vi "Update_Results_file_copies.vi"(2 "Raw data option":enum16{"Save raw data", "Raw data not saved"}(ring), 4 "Raw data file":path, 5 "Results file":path) -> ()   [LabVIEW 2022 SP3]
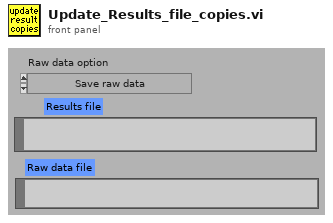
[diagram p1: front panel]
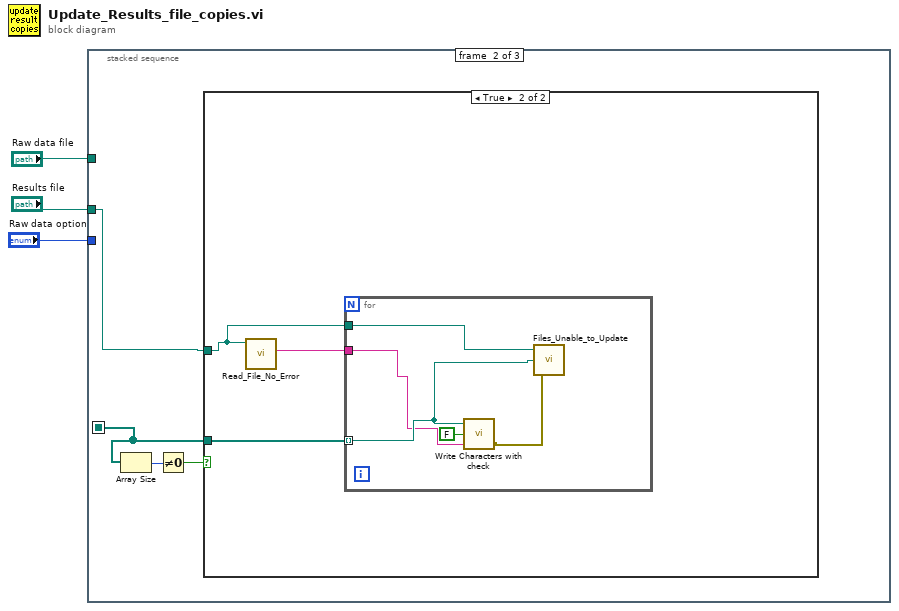
[diagram p0: block diagram]
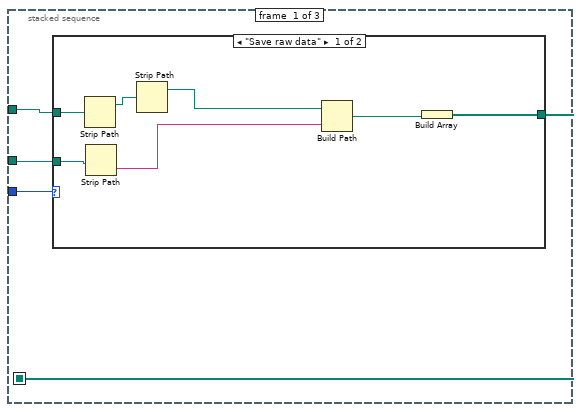
[diagram p2: hidden frame]
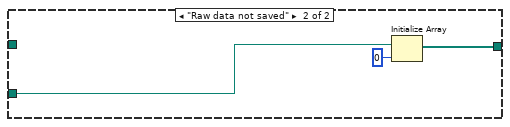
[diagram p3: hidden frame]
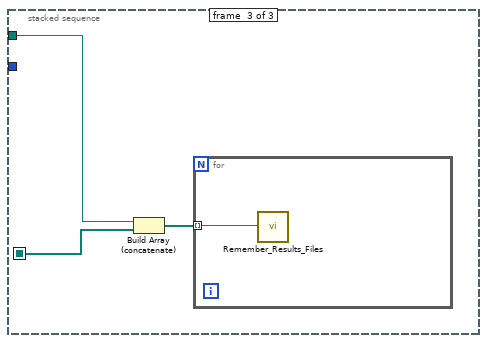
[diagram p5: hidden frame]
diagram:
  n1 = stacked-sequence {
    seq-local: [w4 _ _] -> [_ w18 w30]
    tunnel: "Results file" -> [w7 w19 w31]
    tunnel: "Raw data file" -> [w6 _ _]
    tunnel: "Raw data option" -> [w5 _ _]
    frame #0 {
      n2 = case shown="\"Save raw data\"" w5 {
        tunnel: w6 -> [w12 _]
        tunnel: w7 -> [w13 w15]
        tunnel: [w14 w16] -> w4
        frame "Save raw data" {
          n3 = Strip Path(path=w12) -> (stripped path=w9:path)  [unwired: 1 out]
          n4 = Strip Path(path=w13) -> (name=w11:string)  [unwired: 1 out]
          n5 = Strip Path(path=w9) -> (stripped path=w8:path)  [unwired: 1 out]
          n6 = Build Path(base path=w8, name or relative path=w11) -> (appended path=w10:path)
          n7 = Build Array(w10) -> (w14:path[])
        }
        frame "Raw data not saved" {
          n8 = Initialize Array(w15, 0 ("Dimension Size")) -> (w16:path[])
        }
      }
    }
    frame #1 {
      n9 = Array Size(array=w18) -> (size(s)=w21:i32)
      n10 = Not Equal To 0?(x=w21) -> (x != 0?=w20:bool)
      n11 = case shown="True" w20 {
        tunnel: w19 -> [_ w22]
        tunnel: w18 -> [_ w24]
        frame False {
        }
        frame True {
          n12 = call "Read_File_No_Error.vi"("Filename"=w22) -> ("string"=w23:string)  [unwired: 2 in, 7 out]
          n13 = for {
            tunnel: w24 -> [w28] mode=indexing
            tunnel: w23 -> [w27]
            tunnel: w22 -> [w29]
            n14 = call "Write Characters with check.vi"("String to Write"=w27, "Call EnFlo Error Handler?"=FALSE, "file (use dialog)"=w28) -> ("error out"=w26:errorcluster)  [unwired: 1 in]
            n15 = call "Files_Unable_to_Update.vi"("error in (no error)"=w26, "Target Path"=w28, "Source Path"=w29) -> ()  [unwired: 1 out]
          }
        }
      }
    }
    frame #2 {
      n16 = Build Array (concatenate)(w31, w30) -> (w32:path[])
      n17 = for {
        tunnel: w32 -> [w33] mode=indexing
        n18 = call "Remember_Results_Files.vi"("Filename to Remember"=w33) -> ()  [unwired: 1 out]
      }
    }
  }
